vi "GetTelemValues.vi"(7 "Not Found Value":string="-9999999", 8 "Telemetry In":cluster{"Name":string[], "Value":string[]}, 11 "Telemetry Names":string[](array[string])) -> (0 "Telemetry Out":cluster{"Name":string[], "Value":string[]}, 3 "Telemetry Values":string[](array[string]))   [LabVIEW 2014]
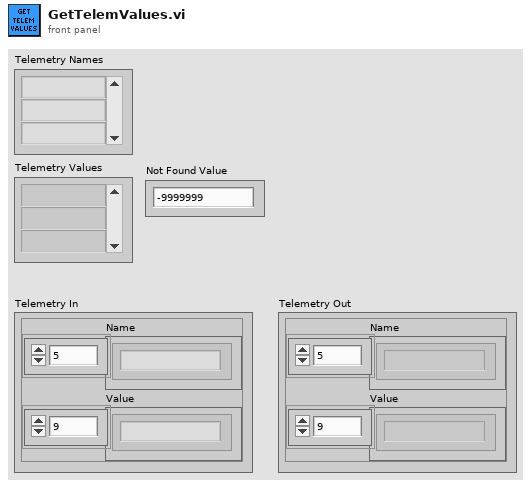
[diagram p1: front panel]
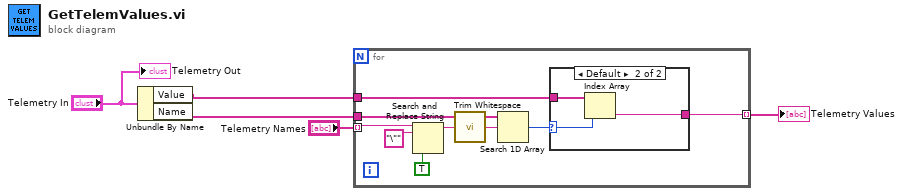
[diagram p0: block diagram]
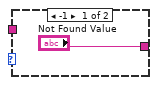
[diagram p2: hidden frame]
diagram:
  n1 = Unbundle By Name("Telemetry In") -> ("Value"=w2:string[], "Name"=w3:string[])
  n2 = for {
    tunnel: "Telemetry Names" -> [w11] mode=indexing
    tunnel: w3 -> [w14]
    tunnel: w2 -> [w13]
    tunnel: [w12] -> w4 mode=indexing
    n3 = Search and Replace String(replace all?=TRUE ("replace all? (F)"), input string=w11, search string="\"") -> (result string=w8:string)  [unwired: 5 in, 3 out]
    n4 = call <vilib>:"Trim Whitespace.vi"("string"=w8) -> ("trimmed string"=w7:string)  [unwired: 1 in]
    n5 = Search 1D Array(1D array=w14, element=w7) -> (index of element=w6:i32)  [unwired: 1 in]
    n6 = case shown="Default" w6 {
      selector: w6 -> [_ w16]
      tunnel: w13 -> [_ w18]
      tunnel: ["Not Found Value" w17] -> w12
      frame -1 {
      }
      frame Default {
        n7 = Index Array(array=w18, index=w16) -> (element=w17:string)
      }
    }
  }
  "Telemetry Values" <- w4
  "Telemetry Out" <- "Telemetry In"
